vi "Divide Vector by Scalar.vi"(1 "Vector":T1 format="%_8f", 4 "x":dbl format="%_8f") -> (15 "Scaled Vector":T1 format="%_8f")   [LabVIEW 2014]
uses:
  <vilib>/Analysis/Matrix/Datatypes/RealMatrix.ctl
  <vilib>/Analysis/Matrix/NI_Matrix.lvlib
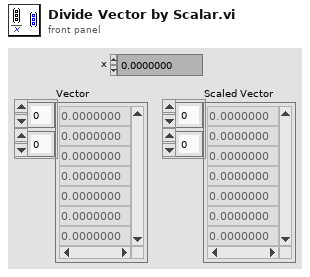
[diagram p1: front panel]
types:
  T1 = typedef "NI_Matrix.lvlib/RealMatrix.ctl" = dbl[][]
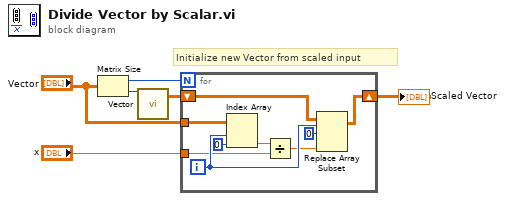
[diagram p0: block diagram]
diagram:
  # "Initialize new Vector from scaled input"
  n1 = Matrix Size(0:"Vector") -> (1:w4:i32, 2:w1:i32)
  n2 = call "Vector.vi"("length"=w1) -> ("Real Matrix (Column Vector)"=w2:T1)  [unwired: 18 in]
  n3 = for {
    N: w4 -> [_]
    tunnel: "Vector" -> [w12]
    shift-right: [w14] -> w3
    shift-left: w2 -> [w15]
    tunnel: "x" -> [w7]
    i -> [w11]
    n4 = Index Array(array=w12, index (row)=w11, index (col)=0) -> (element=w8:dbl)
    n5 = Divide(x=w8, y=w7) -> (x/y=w9:dbl)
    n6 = Replace Array Subset(array=w15, new element=w9, index (row)=w11, index (col)=0 ("disabled index (col)")) -> (w14:T1)
  }
  "Scaled Vector" <- w3
